vi "Find Plots.vi"(9 "Start":cluster{i32, i32}, 10 "Map":map{cluster{i32, i32}, cluster{bool, u64}}(c390), 11 "Steps":i32) -> (3 "Answer":u64)   [LabVIEW 2023, in "d21.lvlib"]
uses:
  d21.lvlib
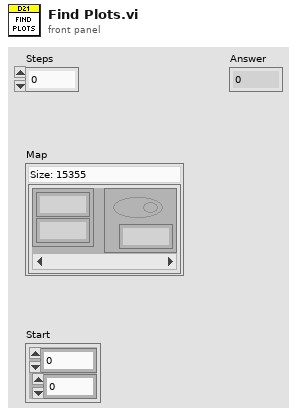
[diagram p1: front panel]
types:
  T1 = cluster{cluster{bool, "f":i32}, "Start":cluster{i32, i32}}
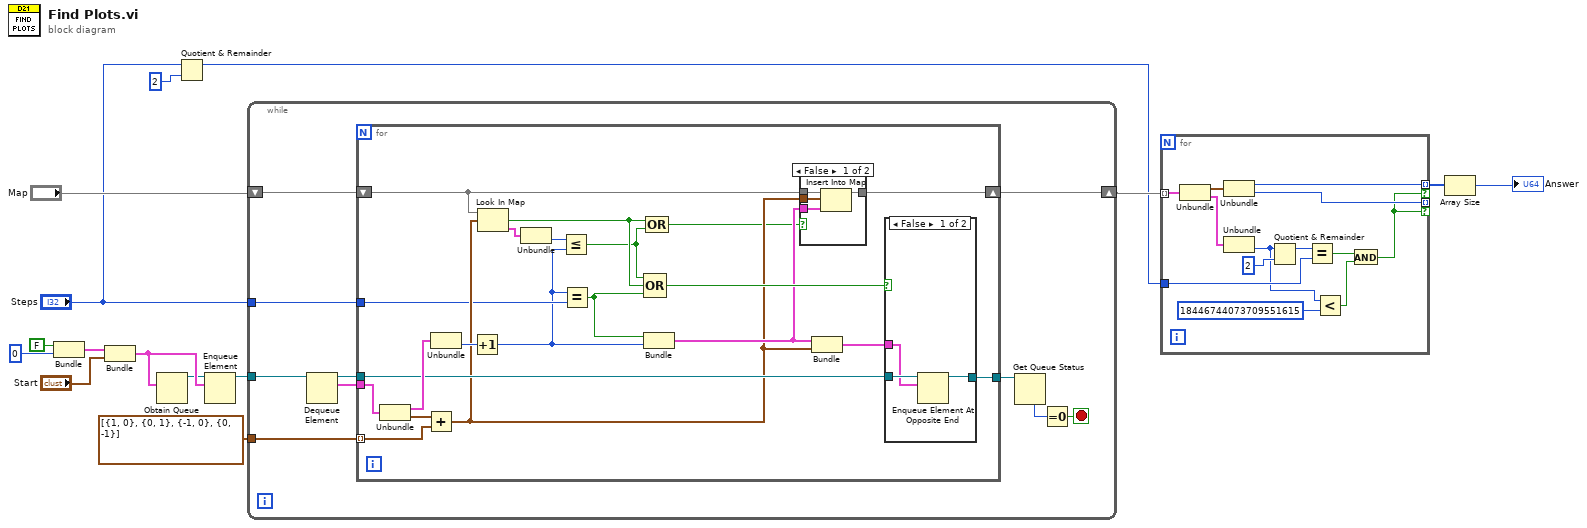
[diagram p0: block diagram]
diagram:
  n1 = Bundle(FALSE, "f"=0) -> (w13:cluster{bool, "f":i32})  [unwired: 1 in]
  n2 = Bundle(w13, "Start"="Start") -> (w12:T1)  [unwired: 1 in]
  n3 = Obtain Queue(element data type=w12) -> (queue out=w7:refnum<queue>)  [unwired: 4 in, 2 out]
  n4 = Quotient & Remainder(x="Steps", y=u64 2) -> (x-y*floor(x/y)=w1:u64)  [unwired: 1 out]
  n5 = Enqueue Element(queue=w7, element=w12) -> (queue out=w8:refnum<queue>)  [unwired: 2 in, 2 out]
  n6 = while {
    tunnel: w8 -> [w24]
    shift-right: [w23] -> w4
    shift-left: "Map" -> [w25]
    tunnel: cluster{i32, i32}[] [{1, 0}, {0, 1}, {-1, 0}, {0, -1}] -> [w22]
    tunnel: "Steps" -> [w16]
    stop <- w17 stop-if-true
    n7 = Dequeue Element(queue=w24) -> (queue out=w20:refnum<queue>, element=w21:T1)  [unwired: 2 in, 2 out]
    n8 = for {
      shift-right: [w35] -> w23
      shift-left: w25 -> [w36]
      tunnel: w22 -> [w46] mode=indexing
      tunnel: w21 -> [w45]
      tunnel: w20 -> [w41]
      tunnel: [w40] -> w19
      tunnel: w16 -> [w28]
      n9 = Unbundle(w45) -> (w42:cluster{bool, "f":i32}, "Start"=w43:cluster{i32, i32})
      n10 = Add(x=w43, y=w46) -> (x+y=w32:cluster{i32, i32})
      n11 = Unbundle(w42) -> ("f"=w44:i32)  [unwired: 1 out]
      n12 = Increment(x=w44) -> (x+1=w27:i32)
      n13 = Look In Map(map=w36, key=w32) -> (key not found?=w37:bool, value=w38:cluster{bool, u64})  [unwired: 1 in]
      n14 = Unbundle(w38) -> (w31:u64)  [unwired: 1 out]
      n15 = Less Or Equal?(x=w31, y=w27) -> (x <= y?=w30:bool)
      n16 = Equal?(x=w27, y=w28) -> (x = y?=w26:bool)
      n17 = Compound Arithmetic op=OR(w30, w37, w26) -> (w39:bool)
      n18 = Bundle(w26, w27) -> (w33:cluster{bool, i32})  [unwired: 1 in]
      n19 = Compound Arithmetic op=OR(w37, w30) -> (w29:bool)
      n20 = case shown="False" w29 {
        tunnel: w36 -> [w50 w51]
        tunnel: [w49 w51] -> w35
        tunnel: w33 -> [w48 _]
        tunnel: w32 -> [w47 _]
        frame False {
          n21 = Insert Into Map(map in=w50, key=w47, value=w48) -> (map out=w49:map{cluster{i32, i32}, cluster{bool, u64}})  [unwired: 2 out]
        }
        frame True {
        }
      }
      n22 = Bundle(w33, w32) -> (w34:cluster{cluster{bool, i32}, cluster{i32, i32}})  [unwired: 1 in]
      n23 = case shown="False" w39 {
        tunnel: w41 -> [w54 w55]
        tunnel: w34 -> [w52 _]
        tunnel: [w53 w55] -> w40
        frame False {
          n24 = Enqueue Element At Opposite End(queue=w54, element=w52) -> (queue out=w53:refnum<queue>)  [unwired: 2 in, 2 out]
        }
        frame True {
        }
      }
    }
    n25 = Get Queue Status(queue=w19) -> (# elements in queue=w18:i32)  [unwired: 2 in, 7 out]
    n26 = Equal To 0?(x=w18) -> (x = 0?=w17:bool)
  }
  n27 = for {
    tunnel: w4 -> [w68] mode=indexing
    tunnel: [w65] -> w6 mode=indexing if=w58
    tunnel: [w64] -> _ mode=indexing if=w58
    tunnel: w1 -> [w60]
    n28 = Unbundle(w68) -> ("output cluster"=w67:cluster{i32, i32}, "output cluster"=w66:cluster{bool, u64})
    n29 = Unbundle(w67) -> (w65:i32, w64:i32)
    n30 = Unbundle(w66) -> (w56:u64)  [unwired: 1 out]
    n31 = Quotient & Remainder(x=w56, y=u64 2) -> (x-y*floor(x/y)=w62:u64)  [unwired: 1 out]
    n32 = Equal?(x=w62, y=w60) -> (x = y?=w59:bool)
    n33 = Less?(x=w56, y=u64 18446744073709551615) -> (x < y?=w61:bool)
    n34 = And(x=w59, y=w61) -> (x .and. y?=w58:bool)
  }
  n35 = Array Size(array=w6) -> (size(s)=→"Answer":i32)
